vi "Setpoint.vi"(8 "error in (no error)":errorcluster, 10 "Setpoint [A]":dbl format="%.5f", 11 "PS Driver AMI4xx.lvlib:PS Driver AMI4xx.lvclass in":refnum<class "PS Driver AMI4xx.lvclass">) -> (0 "error out":errorcluster, 2 "Setpoint out (A)":dbl, 3 "PS Driver AMI4xx.lvlib:PS Driver AMI4xx.lvclass out":refnum<class "PS Driver AMI4xx.lvclass">)   [LabVIEW 2020, in "PS Driver.lvlib" / "PS Driver AMI4xx.lvclass"]
uses:
  PS Driver AMI4xx.lvclass
  PS Driver with Persistence.lvclass
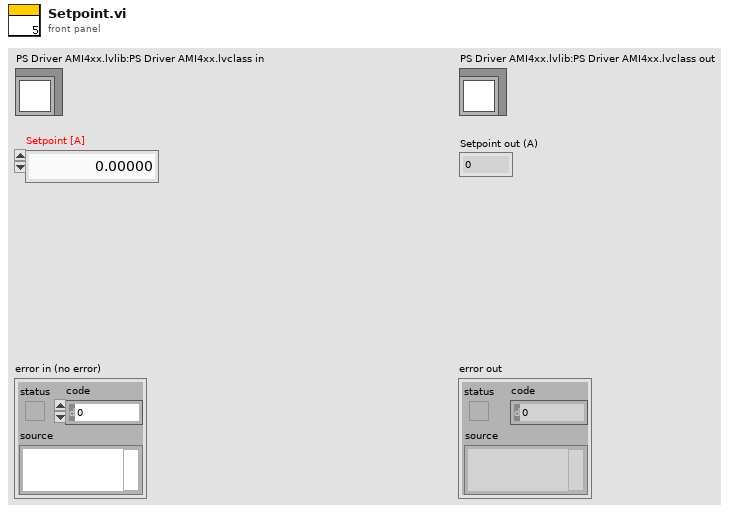
[diagram p1: front panel]
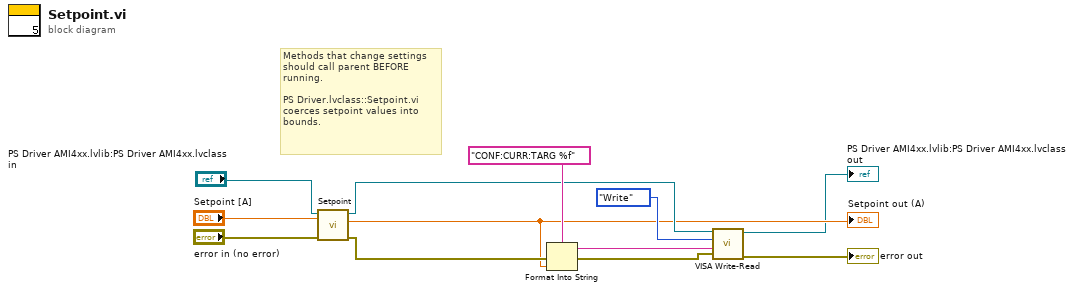
[diagram p0: block diagram]
diagram:
  # "Methods that change settings\nshould call parent BEFORE\nrunning.\n\nPS Driver.lvclass::Setpoint.vi \ncoerces setpoint values into\nbounds."
  n1 = call-parent "Setpoint.vi"("error in (no error)"="error in (no error)", "Setpoint [A]"="Setpoint [A]", "PS Driver.lvlib:PS Driver.lvclass in"="PS Driver AMI4xx.lvlib:PS Driver AMI4xx.lvclass in") -> ("error out"=w5:errorcluster, "Setpoint out (A)"=w2:dbl, "PS Driver.lvlib:PS Driver.lvclass out"=w7:refnum<class "PS Driver AMI4xx.lvclass">)  [unwired: 6 in]
  "Setpoint out (A)" <- w2
  n2 = Format Into String(format string="CONF:CURR:TARG %f" ("Command String"), error in=w5, w2) -> (resulting string=w10:string, error out=w4:errorcluster)  [unwired: 1 in]
  n3 = call "VISA Write-Read.vi"("error in (no error)"=w4, "Command String"=w10, "Action"=enum16{"Write", "Read", "Write & Read"}."Write", "PS Driver.lvlib:PS Driver AMI4xx.lvclass"=w7) -> ("error out"=→"error out":errorcluster, "PS Driver.lvlib:PS Driver AMI4xx.lvclass out"=→"PS Driver AMI4xx.lvlib:PS Driver AMI4xx.lvclass out":refnum<class "PS Driver AMI4xx.lvclass">)  [unwired: 4 in, 2 out]
